vi "Calculate Vertex Array.vi"(8 "error in (no error)":errorcluster, 9 "Coordinates System":enum16{"Cartesian", "Cylindrical", "Spherical"}(ring)=enum."Spherical", 10 "3D Comet Datatype.lvclass in":refnum<class "3D Comet Datatype.lvclass">, 11 "Plot Representation In":T1) -> (0 "error out":errorcluster, 1 "Dup Coordinates System":enum16{"Cartesian", "Cylindrical", "Spherical"}(ring)=enum."Spherical", 2 "3D Comet Datatype.lvclass out":refnum<class "3D Comet Datatype.lvclass">, 3 "Plot Representation Out":T1)   [LabVIEW 2017, in "3D Comet Datatype.lvclass"]
uses:
  <vilib>/Math Plots/3D Math Plots/3D Comet/3D Comet Datatype/3D Comet Datatype.lvclass
  <vilib>/Math Plots/3D Math Plots/3D Plot/3D Plot/Typedef/Plot Representation.ctl
  <vilib>/Math Plots/3D Math Plots/3D Plot/3D Plot/Typedef/Range Clusters.ctl
  <vilib>/Math Plots/3D Math Plots/3D Plot/3D Plot/Typedef/Mesh Data.ctl
  <vilib>/Math Plots/3D Math Plots/3D Comet/3D Comet Datatype/3D Comet Datatype.lvclass/3D Comet Datatype.ctl
  <vilib>/Math Plots/3D Math Plots/3D Plot/3D Plot Datatype/3D Plot Datatype.lvclass
  <vilib>/Math Plots/3D Math Plots/3D Plot/3D Plot/3D Plot.lvclass
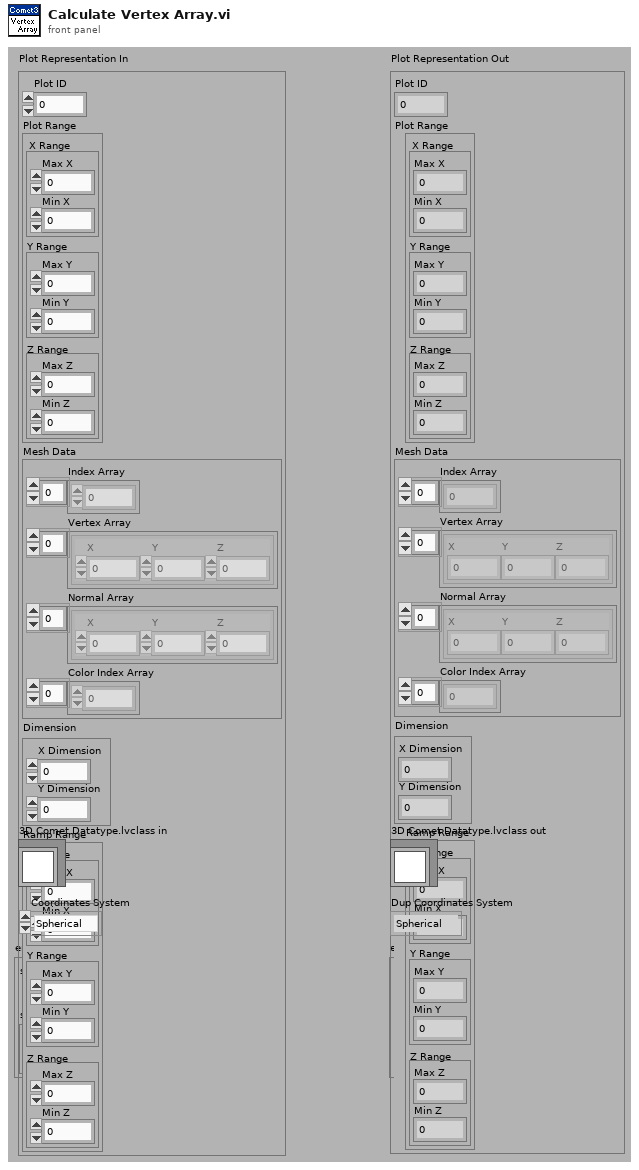
[diagram p1: front panel]
types:
  T1 = typedef "3D Plot.lvclass/Plot Representation.ctl" = cluster{"Plot ID":i32, "Plot Range":T2, "Mesh Data":T3, "Dimension":cluster{"X Dimension":i32, "Y Dimension":i32}, "Ramp Range":T2}
  T2 = typedef "3D Plot.lvclass/Range Clusters.ctl" = cluster{"X Range":cluster{"Max X":sgl, "Min X":sgl}, "Y Range":cluster{"Max Y":sgl, "Min Y":sgl}, "Z Range":cluster{"Max Z":sgl, "Min Z":sgl}}
  T3 = typedef "3D Plot.lvclass/Mesh Data.ctl" = cluster{"Index Array":u32[], "Vertex Array":cluster{"X":sgl, "Y":sgl, "Z":sgl}[], "Normal Array":cluster{"X":sgl, "Y":sgl, "Z":sgl}[], "Color Index Array":i32[]}
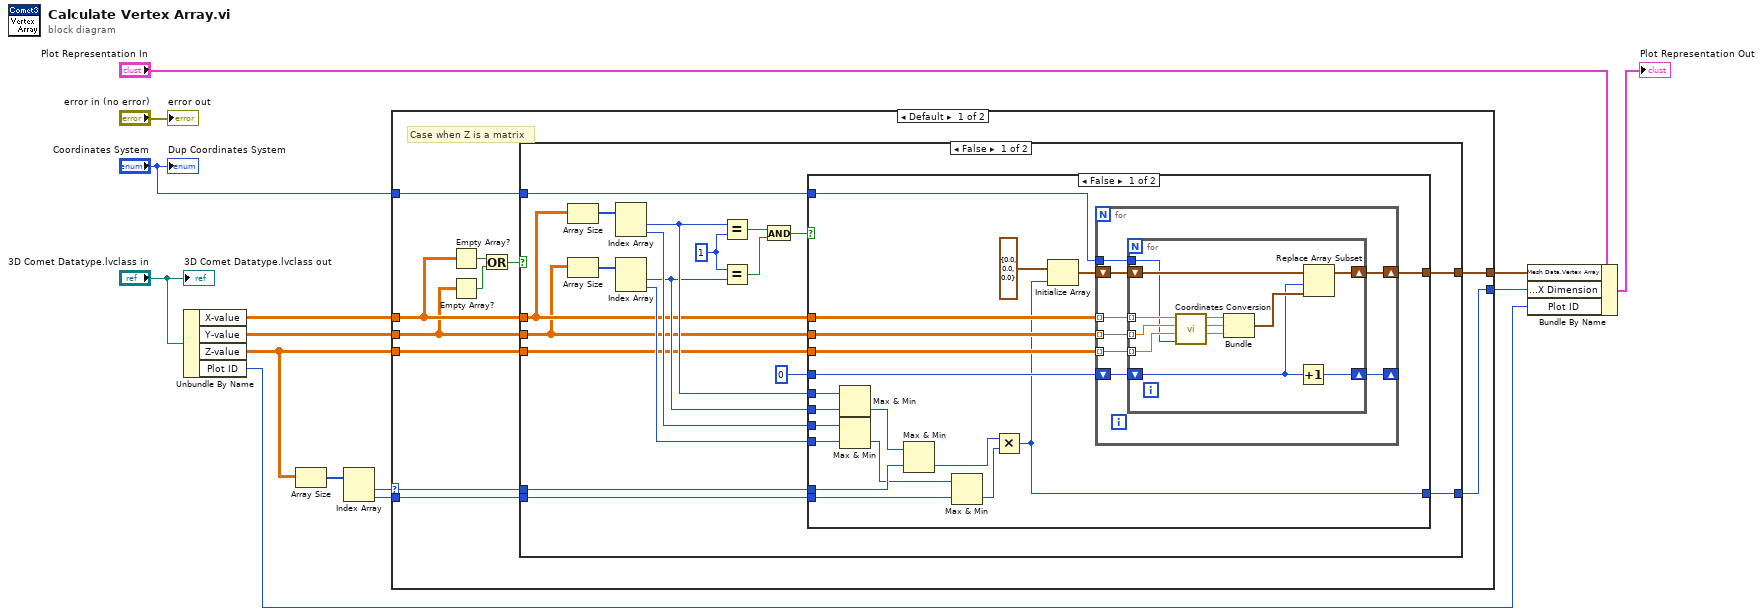
[diagram p0: block diagram]
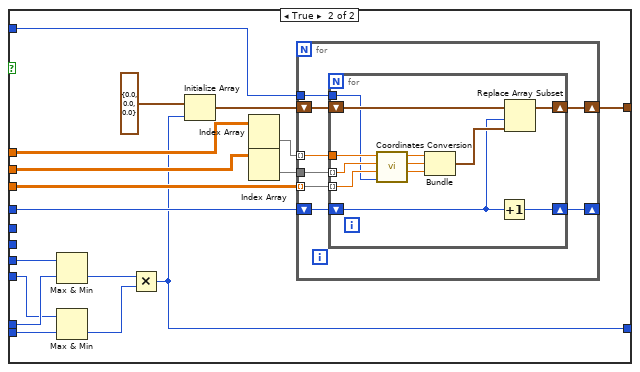
[diagram p2: hidden frame]
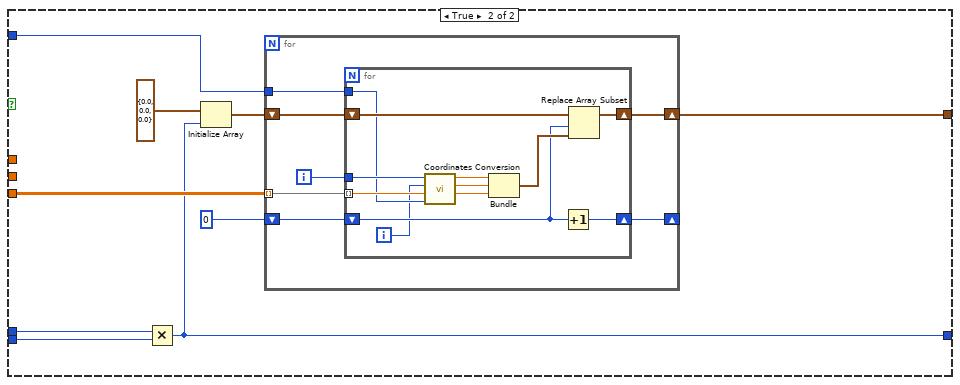
[diagram p3: hidden frame]
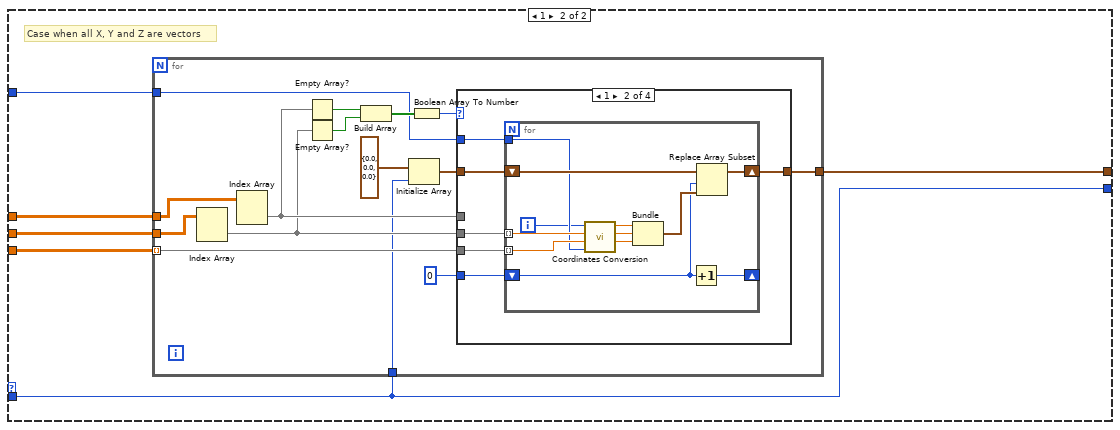
[diagram p4: hidden frame]
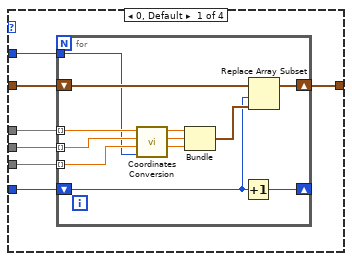
[diagram p5: hidden frame]
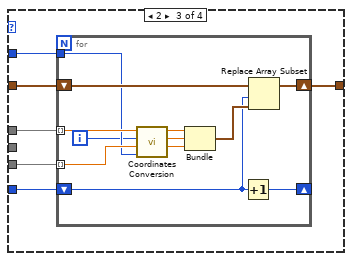
[diagram p6: hidden frame]
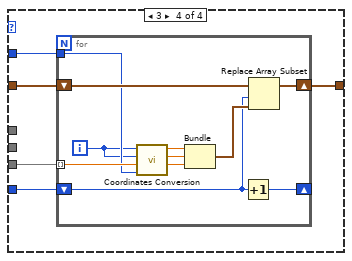
[diagram p7: hidden frame]
diagram:
  n1 = Unbundle By Name("3D Comet Datatype.lvclass in") -> ("X-value"=w1:sgl[][], "Y-value"=w2:sgl[][], "Z-value"=w6:sgl[][], "Plot ID"=w13:i32)
  n2 = Array Size(array=w6) -> (size(s)=w12:i32[])
  n3 = Index Array(array=w12) -> (element #1=w8:i32, element #2=w7:i32)  [unwired: 2 in]
  n4 = case shown="Default" w8 {
    selector: w8 -> [w18 _]
    tunnel: w1 -> [w21 w154]
    tunnel: w2 -> [w20 w153]
    tunnel: w6 -> [w19 w152]
    tunnel: "Coordinates System" -> [w25 w151]
    tunnel: w7 -> [w17 w149]
    tunnel: [w16 w149] -> w3
    tunnel: [w15 w150] -> w4
    frame Default {
      # "Case when Z is a matrix"
      n5 = Empty Array?(array=w21) -> (empty?=w23:bool)
      n6 = Empty Array?(array=w20) -> (empty?=w24:bool)
      n7 = Or(x=w23, y=w24) -> (x .or. y?=w22:bool)
      n8 = case shown="False" w22 {
        tunnel: [w27 w129] -> w15
        tunnel: w18 -> [w29 w123]
        tunnel: w19 -> [w30 w128]
        tunnel: w25 -> [w33 w127]
        tunnel: [w26 w121] -> w16
        tunnel: w21 -> [w32 _]
        tunnel: w20 -> [w31 _]
        tunnel: w17 -> [w28 w122]
        frame False {
          w42 = 1 ("x")
          n9 = Array Size(array=w32) -> (size(s)=w44:i32[])
          n10 = Array Size(array=w31) -> (size(s)=w43:i32[])
          n11 = Index Array(array=w44) -> (element #1=w35:i32, element #2=w37:i32)  [unwired: 2 in]
          n12 = Index Array(array=w43) -> (element #1=w34:i32, element #2=w36:i32)  [unwired: 2 in]
          n13 = Equal?(x=w35, y=w42) -> (x = y?=w41:bool)
          n14 = Equal?(x=w42, y=w34) -> (x = y?=w40:bool)
          n15 = And(x=w41, y=w40) -> (x .and. y?=w39:bool)
          n16 = case shown="False" w39 {
            tunnel: w33 -> [w63 w100]
            tunnel: w32 -> [w62 w96]
            tunnel: w31 -> [w61 w95]
            tunnel: w30 -> [w60 w97]
            tunnel: 0 -> [w59 w98]
            tunnel: [w58 w99] -> w27
            tunnel: w37 -> [w53 w90]
            tunnel: w29 -> [w50 w89]
            tunnel: w36 -> [w52 w88]
            tunnel: w28 -> [w48 w87]
            tunnel: [w45 w84] -> w26
            tunnel: w35 -> [w55 _]
            tunnel: w34 -> [w54 _]
            frame False {
              n17 = Max & Min(x=w55, y=w54) -> (min(x,y)=w51:i32)  [unwired: 1 out]
              n18 = Max & Min(x=w53, y=w52) -> (min(x,y)=w49:i32)  [unwired: 1 out]
              n19 = Max & Min(x=w51, y=w50) -> (min(x,y)=w47:i32)  [unwired: 1 out]
              n20 = Max & Min(x=w49, y=w48) -> (min(x,y)=w46:i32)  [unwired: 1 out]
              n21 = Multiply(x=w47, y=w46) -> (x*y=w45:i32)
              n22 = Initialize Array(cluster{"X":sgl, "Y":sgl, "Z":sgl} {"X"=0.0, "Y"=0.0, "Z"=0.0} ("3D Point"), w45) -> (w56:cluster{"X":sgl, "Y":sgl, "Z":sgl}[])
              n23 = for {
                shift-right: [w70] -> w58
                shift-left: w56 -> [w71]
                tunnel: w60 -> [w69] mode=indexing
                tunnel: w62 -> [w67] mode=indexing
                tunnel: w61 -> [w68] mode=indexing
                tunnel: w63 -> [w66]
                shift-right: [w64] -> _
                shift-left: w59 -> [w65]
                n24 = for {
                  tunnel: w69 -> [w79] mode=indexing
                  shift-right: [w83] -> w70
                  shift-left: w71 -> [w82]
                  tunnel: w68 -> [w80] mode=indexing
                  tunnel: w67 -> [w81] mode=indexing
                  tunnel: w66 -> [w75]
                  shift-right: [w73] -> w64
                  shift-left: w65 -> [w72]
                  n25 = call <vilib>:"Coordinates Conversion.vi"("Coordinates System"=w75, "Z in"=w79, "Y in"=w80, "X in"=w81) -> ("Z out"=w76:sgl, "Y out"=w77:sgl, "X out"=w78:sgl)  [unwired: 5 out]
                  n26 = Bundle("X out"=w78, "Y out"=w77, "Z out"=w76) -> (w74:cluster{"X out":sgl, "Y out":sgl, "Z out":sgl})  [unwired: 1 out]
                  n27 = Increment(x=w72) -> (x+1=w73:i32)
                  n28 = Replace Array Subset(array=w82, new element=w74, index=w72) -> (w83:cluster{"X":sgl, "Y":sgl, "Z":sgl}[])
                }
              }
            }
            frame True {
              n29 = Max & Min(x=w90, y=w89) -> (min(x,y)=w86:i32)  [unwired: 1 out]
              n30 = Max & Min(x=w88, y=w87) -> (min(x,y)=w85:i32)  [unwired: 1 out]
              n31 = Multiply(x=w86, y=w85) -> (x*y=w84:i32)
              n32 = Initialize Array(cluster{"X":sgl, "Y":sgl, "Z":sgl} {"X"=0.0, "Y"=0.0, "Z"=0.0} ("3D Point"), w84) -> (w91:cluster{"X":sgl, "Y":sgl, "Z":sgl}[])
              n33 = Index Array(array=w96) -> (element=w93:sgl[])  [unwired: 2 in]
              n34 = Index Array(array=w95) -> (element=w94:sgl[])  [unwired: 2 in]
              n35 = for {
                shift-right: [w107] -> w99
                shift-left: w91 -> [w108]
                tunnel: w97 -> [w106] mode=indexing
                tunnel: w93 -> [w104] mode=indexing
                tunnel: w94 -> [w105]
                tunnel: w100 -> [w103]
                shift-right: [w101] -> _
                shift-left: w98 -> [w102]
                n36 = for {
                  tunnel: w106 -> [w116] mode=indexing
                  shift-right: [w120] -> w107
                  shift-left: w108 -> [w119]
                  tunnel: w105 -> [w117] mode=indexing
                  tunnel: w104 -> [w118]
                  tunnel: w103 -> [w112]
                  shift-right: [w110] -> w101
                  shift-left: w102 -> [w109]
                  n37 = call <vilib>:"Coordinates Conversion.vi"("Coordinates System"=w112, "Z in"=w116, "Y in"=w117, "X in"=w118) -> ("Z out"=w113:sgl, "Y out"=w114:sgl, "X out"=w115:sgl)  [unwired: 5 out]
                  n38 = Bundle("X out"=w115, "Y out"=w114, "Z out"=w113) -> (w111:cluster{"X out":sgl, "Y out":sgl, "Z out":sgl})  [unwired: 1 out]
                  n39 = Increment(x=w109) -> (x+1=w110:i32)
                  n40 = Replace Array Subset(array=w119, new element=w111, index=w109) -> (w120:cluster{"X":sgl, "Y":sgl, "Z":sgl}[])
                }
              }
            }
          }
        }
        frame True {
          n41 = Multiply(x=w123, y=w122) -> (x*y=w121:i32)
          n42 = Initialize Array(cluster{"X":sgl, "Y":sgl, "Z":sgl} {"X"=0.0, "Y"=0.0, "Z"=0.0} ("3D Point"), w121) -> (w125:cluster{"X":sgl, "Y":sgl, "Z":sgl}[])
          n43 = for {
            shift-right: [w135] -> w129
            shift-left: w125 -> [w136]
            tunnel: w128 -> [w134] mode=indexing
            tunnel: w127 -> [w133]
            shift-right: [w131] -> _
            shift-left: 0 -> [w132]
            i -> [w130]
            n44 = for {
              tunnel: w134 -> [w145] mode=indexing
              shift-right: [w148] -> w135
              shift-left: w136 -> [w147]
              tunnel: w130 -> [w146]
              tunnel: w133 -> [w141]
              shift-right: [w139] -> w131
              shift-left: w132 -> [w138]
              i -> [w137]
              n45 = call <vilib>:"Coordinates Conversion.vi"("Coordinates System"=w141, "Z in"=w145, "Y in"=w137, "X in"=w146) -> ("Z out"=w142:sgl, "Y out"=w143:sgl, "X out"=w144:sgl)  [unwired: 5 out]
              n46 = Bundle("X out"=w144, "Y out"=w143, "Z out"=w142) -> (w140:cluster{"X out":sgl, "Y out":sgl, "Z out":sgl})  [unwired: 1 out]
              n47 = Increment(x=w138) -> (x+1=w139:i32)
              n48 = Replace Array Subset(array=w147, new element=w140, index=w138) -> (w148:cluster{"X":sgl, "Y":sgl, "Z":sgl}[])
            }
          }
        }
      }
    }
    frame 1 {
      # "Case when all X, Y and Z are vectors"
      n49 = for {
        tunnel: w154 -> [w159]
        tunnel: w153 -> [w158]
        tunnel: w152 -> [w162] mode=indexing
        tunnel: w151 -> [w161]
        tunnel: [w160] -> w150
        tunnel: w149 -> [w155]
        n50 = Index Array(array=w158) -> (element=w156:sgl[])  [unwired: 2 in]
        n51 = Index Array(array=w159) -> (element=w157:sgl[])  [unwired: 2 in]
        n52 = Empty Array?(array=w157) -> (empty?=w164:bool)
        n53 = Empty Array?(array=w156) -> (empty?=w165:bool)
        n54 = Build Array(w164, w165) -> (w166:bool[])
        n55 = Initialize Array(cluster{"X":sgl, "Y":sgl, "Z":sgl} {"X"=0.0, "Y"=0.0, "Z"=0.0} ("3D Point"), w155) -> (w168:cluster{"X":sgl, "Y":sgl, "Z":sgl}[])
        n56 = Boolean Array To Number(Boolean array=w166) -> (number=w163:u32)
        n57 = case shown="1" w163 {
          tunnel: [w176 w194 w212 w229] -> w160
          tunnel: w168 -> [w175 w193 w211 w228]
          tunnel: 0 -> [w174 w192 w210 w227]
          tunnel: w162 -> [w173 w191 w209 w226]
          tunnel: w157 -> [w172 _ w208 _]
          tunnel: w156 -> [w171 w190 _ _]
          tunnel: w161 -> [w170 w189 w207 w225]
          frame 0, Default {
            n58 = for {
              shift-right: [w187] -> w176
              shift-left: w175 -> [w188]
              tunnel: w173 -> [w184] mode=indexing
              tunnel: w172 -> [w186] mode=indexing
              tunnel: w171 -> [w185] mode=indexing
              tunnel: w170 -> [w180]
              shift-right: [w178] -> _
              shift-left: w174 -> [w177]
              n59 = call <vilib>:"Coordinates Conversion.vi"("Coordinates System"=w180, "Z in"=w184, "Y in"=w185, "X in"=w186) -> ("Z out"=w181:sgl, "Y out"=w182:sgl, "X out"=w183:sgl)  [unwired: 5 out]
              n60 = Bundle("X out"=w183, "Y out"=w182, "Z out"=w181) -> (w179:cluster{"X out":sgl, "Y out":sgl, "Z out":sgl})  [unwired: 1 out]
              n61 = Increment(x=w177) -> (x+1=w178:i32)
              n62 = Replace Array Subset(array=w188, new element=w179, index=w177) -> (w187:cluster{"X":sgl, "Y":sgl, "Z":sgl}[])
            }
          }
          frame 1 {
            n63 = for {
              shift-right: [w205] -> w194
              shift-left: w193 -> [w206]
              tunnel: w191 -> [w203] mode=indexing
              tunnel: w190 -> [w204] mode=indexing
              tunnel: w189 -> [w199]
              shift-right: [w197] -> _
              shift-left: w192 -> [w196]
              i -> [w195]
              n64 = call <vilib>:"Coordinates Conversion.vi"("Coordinates System"=w199, "Z in"=w203, "Y in"=w204, "X in"=w195) -> ("Z out"=w200:sgl, "Y out"=w201:sgl, "X out"=w202:sgl)  [unwired: 5 out]
              n65 = Bundle("X out"=w202, "Y out"=w201, "Z out"=w200) -> (w198:cluster{"X out":sgl, "Y out":sgl, "Z out":sgl})  [unwired: 1 out]
              n66 = Increment(x=w196) -> (x+1=w197:i32)
              n67 = Replace Array Subset(array=w206, new element=w198, index=w196) -> (w205:cluster{"X":sgl, "Y":sgl, "Z":sgl}[])
            }
          }
          frame 2 {
            n68 = for {
              shift-right: [w223] -> w212
              shift-left: w211 -> [w224]
              tunnel: w209 -> [w221] mode=indexing
              tunnel: w208 -> [w222] mode=indexing
              tunnel: w207 -> [w217]
              shift-right: [w215] -> _
              shift-left: w210 -> [w214]
              i -> [w213]
              n69 = call <vilib>:"Coordinates Conversion.vi"("Coordinates System"=w217, "Z in"=w221, "Y in"=w213, "X in"=w222) -> ("Z out"=w218:sgl, "Y out"=w219:sgl, "X out"=w220:sgl)  [unwired: 5 out]
              n70 = Bundle("X out"=w220, "Y out"=w219, "Z out"=w218) -> (w216:cluster{"X out":sgl, "Y out":sgl, "Z out":sgl})  [unwired: 1 out]
              n71 = Increment(x=w214) -> (x+1=w215:i32)
              n72 = Replace Array Subset(array=w224, new element=w216, index=w214) -> (w223:cluster{"X":sgl, "Y":sgl, "Z":sgl}[])
            }
          }
          frame 3 {
            n73 = for {
              shift-right: [w239] -> w229
              shift-left: w228 -> [w240]
              tunnel: w226 -> [w238] mode=indexing
              tunnel: w225 -> [w234]
              shift-right: [w232] -> _
              shift-left: w227 -> [w231]
              i -> [w230]
              n74 = call <vilib>:"Coordinates Conversion.vi"("Coordinates System"=w234, "Z in"=w238, "Y in"=w230, "X in"=w230) -> ("Z out"=w235:sgl, "Y out"=w236:sgl, "X out"=w237:sgl)  [unwired: 5 out]
              n75 = Bundle("X out"=w237, "Y out"=w236, "Z out"=w235) -> (w233:cluster{"X out":sgl, "Y out":sgl, "Z out":sgl})  [unwired: 1 out]
              n76 = Increment(x=w231) -> (x+1=w232:i32)
              n77 = Replace Array Subset(array=w240, new element=w233, index=w231) -> (w239:cluster{"X":sgl, "Y":sgl, "Z":sgl}[])
            }
          }
        }
      }
    }
  }
  n78 = Bundle By Name(cluster="Plot Representation In", "Mesh Data.Vertex Array"=w4, "Dimension.X Dimension"=w3, "Plot ID"=w13) -> (→"Plot Representation Out":T1)
  "error out" <- "error in (no error)"
  "3D Comet Datatype.lvclass out" <- "3D Comet Datatype.lvclass in"
  "Dup Coordinates System" <- "Coordinates System"
